vi "module-09-analog-scale.vi"() -> ()   [LabVIEW 2019]
uses:
  samples-common-library/Ctrl_Training_Library_Protected/CtrlTrainingLibary_Protected.lvlib
panel:
  in  "Tab Control":enum32{"Control Panel", "Logic"}(tab)
  out "Eng Units\nOutput":dbl
  in  "Low Eng Units\nValue":dbl min=-100.0 max=100.0
  in  "Raw Input":dbl=1.25 step=0.05
  out "Calc M":dbl
  out "Trend":cluster{"Raw Input":dbl, "Output":dbl}(graph)
  in  "High Eng Units\nValue":dbl=100.0 min=-100.0 max=100.0
  out "Calc B":dbl
  in  "Low Raw\nValue":dbl min=-100.0 max=100.0
  in  "High Raw\nValue":dbl=5.0 min=-100.0 max=100.0
  # "Analog Value Scaling"
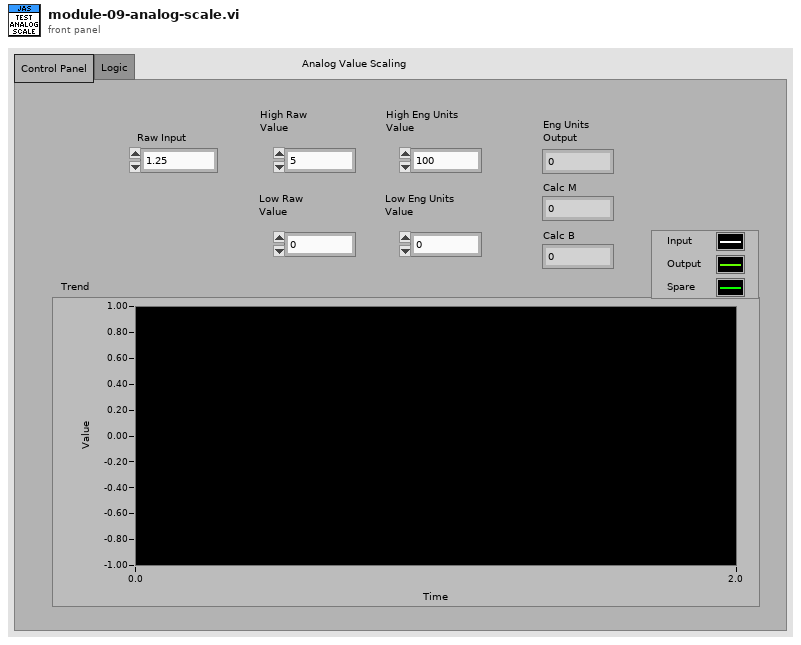
[diagram p1: front panel]
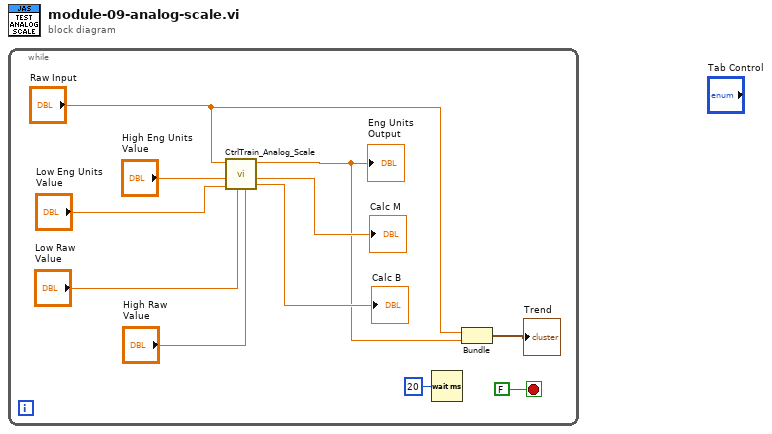
[diagram p0: block diagram]
diagram:
  n1 = while {
    stop <- FALSE stop-if-true
    n2 = call "CtrlTrain_Analog_Scale.vi"("Raw_High"="High Raw\nValue", "Raw_Low"="Low Raw\nValue", "Out_Low"="Low Eng Units\nValue", "Out_High"="High Eng Units\nValue", "Input"="Raw Input") -> ("B"=→"Calc B":dbl, "M"=→"Calc M":dbl, "Output"=w2:dbl)  [unwired: 4 in]
    "Eng Units\nOutput" <- w2
    n3 = Wait (ms)(milliseconds to wait=u32 20) -> ()  [unwired: 1 out]
    n4 = Bundle("Raw Input"="Raw Input", "Output"=w2) -> (→"Trend":cluster{"Raw Input":dbl, "Output":dbl})  [unwired: 1 in]
  }
